vi "GlobalGetTimingsFromCamera.vi"() -> ()   [LabVIEW 2011]
panel:
  in  "Accumulation Camera 1":dbl format="%#_3e"
  in  "Kinetics Camera 1":dbl format="%#_3e"
  in  "Exposure Camera 1":dbl format="%#_3e"
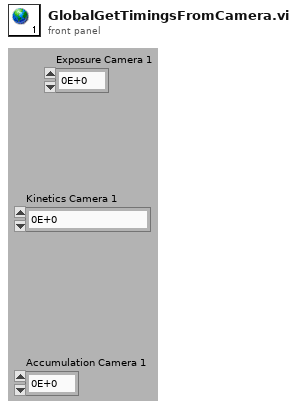
[diagram p1: front panel]
diagram:
